vi "IIR Cascade Filter.vi"   [LabVIEW 2012, in "NI_AALBase.lvlib"]
doc: "Filters the input sequence <B>X</B> using the cascade form of the IIR filter specified by the <B>IIR Filter Cluster</B>. Wire data to the <B>X</B> input to determine the polymorphic instance to use or manually select the instance."
uses:
  NI_AALBase.lvlib
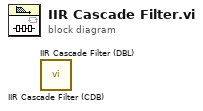
[diagram p0: block diagram]
diagram:
  n1 = call "IIR Cascade Filter (CDB).vi"() -> ()  [unwired: 3 in, 2 out]
  n2 = call "IIR Cascade Filter (DBL).vi"() -> ()  [unwired: 3 in, 2 out]
